vi "DtOLReadMultiple1D.vi"(6 "Buffer size":u32, 7 "OnlyReadAvailable":bool, 8 "error in (no error)":errorcluster, 9 "Timeout":dbl=10.0, 10 "Samples Per Channel":i32=-1, 11 "Task in":i32) -> (0 "error out":errorcluster, 1 "Num Samples Read":u32, 2 "1D Data out":dbl[](array[numeric]), 3 "Task out":i32)   [LabVIEW 2022 SP3]
doc: "Reads multiple samples from a single virtual channel of a task you specify, and returns the data as a one-dimensional array of 32-bit integers. \n\nThis VI is typically used with analog input tasks that use the OLTiming (Input - Set Timing) VI."
uses:
  DtLvLink.lvlib
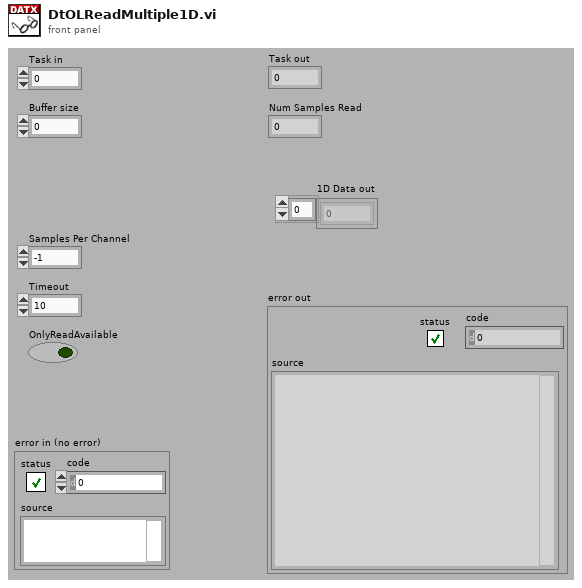
[diagram p1: front panel]
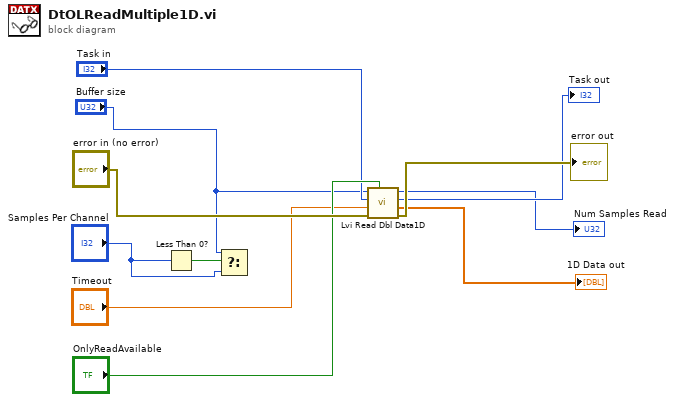
[diagram p0: block diagram]
diagram:
  n1 = Less Than 0?(x="Samples Per Channel") -> (x < 0?=w6:bool)
  n2 = Select(t="Buffer size", s=w6, f="Samples Per Channel") -> ()  [unwired: 1 out]
  n3 = call "Lvi Read Dbl Data1D.vi"("OnlyReadAvailable"="OnlyReadAvailable", "error in (no error)"="error in (no error)", "timeout"="Timeout", "TaskRef"="Task in", "DataBufSize"="Buffer size") -> ("error out"=→"error out":errorcluster, "DataBuf"=→"1D Data out":dbl[], "TaskRef out"=→"Task out":i32, "DataBufSize out"=→"Num Samples Read":u32)  [unwired: 2 in, 1 out]
